vi "Gaussian_fit.vi"(5 "Input waveform":i32[](array[numeric]), 6 "s":bool, 7 "X Values":dbl[](array[numeric])) -> (0 "Gaussian fit":i32[](array[numeric]), 3 "Fit cluster":T1)   [LabVIEW 2019]
uses:
  SiPM_Tests_Global_Var.vi
  <vilib>/Analysis/NI_AALPro.lvlib
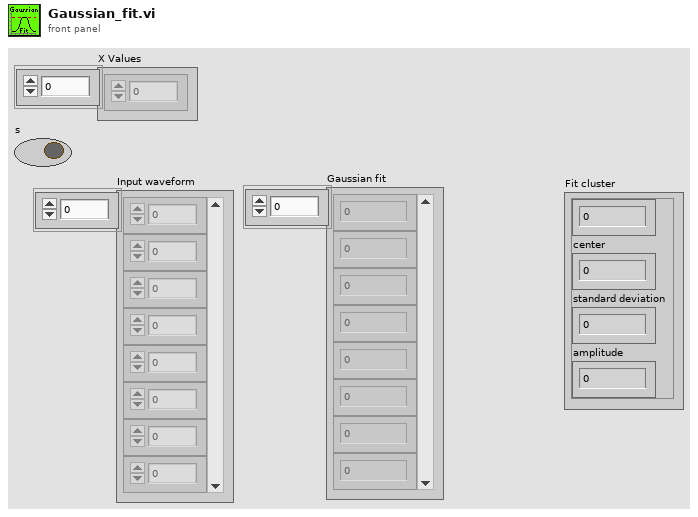
[diagram p1: front panel]
types:
  T1 = cluster{"Numeric Control":dbl, "center":dbl, "standard deviation":dbl, "amplitude":dbl}
  T2 = cluster{"initial amplitude":dbl, "initial center":dbl, "initial standard deviation":dbl, "offset":dbl}
  T3 = typedef "NI_AALPro.lvlib/Curve Fitting Criteria.ctl" = u16
  T4 = cluster{dbl, "center":dbl, "standard deviation":dbl, "amplitude":dbl}
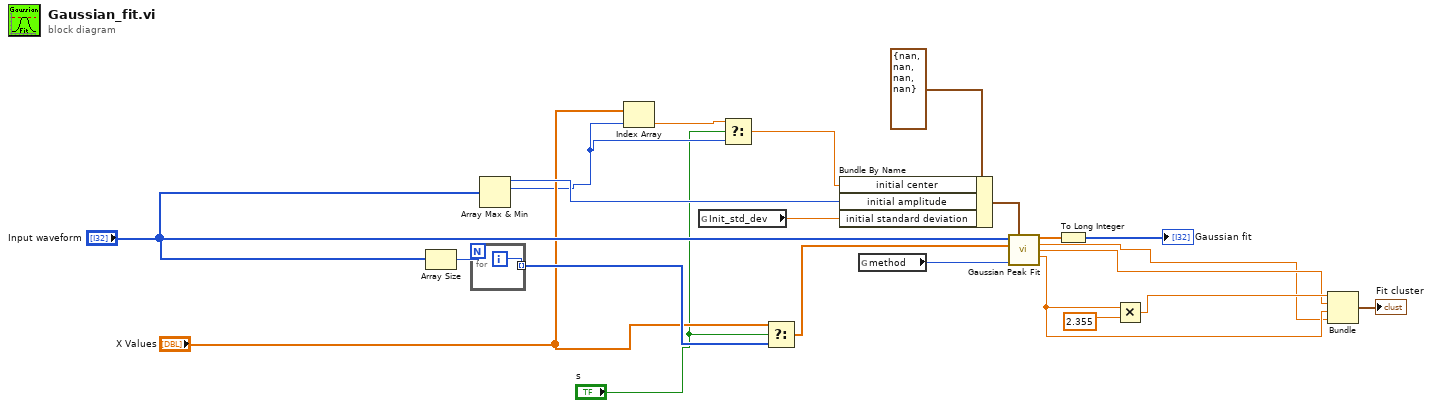
[diagram p0: block diagram]
diagram:
  n1 = Array Size(array="Input waveform") -> (size(s)=w20:i32)
  n2 = for {
    N: w20 -> [_]
    tunnel: [w23] -> w7 mode=indexing
    i -> [w23]
  }
  n3 = Array Max & Min(array="Input waveform") -> (max value=w8:i32, max index (indices)=w3:i32)  [unwired: 2 out]
  n4 = Index Array(array="X Values", index=w3) -> (element=w4:dbl)
  n5 = global read "SiPM_Tests_Global_Var.vi" "Init_std_dev"() -> (w11:dbl)
  n6 = Select(t=w4, s="s", f=w3) -> (s? t:f=w1:dbl)
  n7 = Select(t="X Values", s="s", f=w7) -> (s? t:f=w6:dbl[])
  n8 = Bundle By Name(cluster=T2 {"initial amplitude"=nan, "initial center"=nan, "initial standard deviation"=nan, "offset"=nan} ("initial guess"), "initial center"=w1, "initial amplitude"=w8, "initial standard deviation"=w11) -> (w19:T2)
  n9 = global read "SiPM_Tests_Global_Var.vi" "method"() -> (w10:T3)
  n10 = call <vilib>:"Gaussian Peak Fit.vi"("Y"="Input waveform", "initial guess"=w19, "X"=w6, "method"=w10) -> ("Best Gaussian Fit"=w21:dbl[], "amplitude"=w13:dbl, "center"=w15:dbl, "standard deviation"=w14:dbl)  [unwired: 5 in, 3 out]
  n11 = To Long Integer(number=w21) -> (32bit integer=→"Gaussian fit":i32[])
  n12 = Multiply(x=w14, y=2.355) -> (x*y=w16:dbl)
  n13 = Bundle(w16, "center"=w15, "standard deviation"=w14, "amplitude"=w13) -> (→"Fit cluster":T4)  [unwired: 1 in]
